vi "Offset Structure.vi"(10 "Structure Type":T1, 11 "MasterRect in":T2) -> (3 "MasterRect out":T2)   [LabVIEW 2020, in "Enclose in Structure.lvlib"]
uses:
  Enclose in Structure.lvlib
  <vilib>/Utility/miscctls.llb/LVRectTypeDef.ctl
  Structure Type.ctl
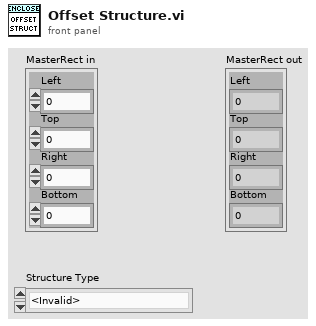
[diagram p1: front panel]
types:
  T1 = typedef "Enclose in Structure.lvlib/Structure Type.ctl" = enum16{"<Invalid>", "For Loop", "While Loop", "Timed Loop", "Timed Sequence", "Case Structure", "Event Structure", "In Place Element Structure", "Flat Sequence", "Diagram Disable Structure", "Conditional Disable Structure", "Type Specialization Structure"}
  T2 = typedef "LVRectTypeDef.ctl" = cluster{"Left":i16, "Top":i16, "Right":i16, "Bottom":i16}
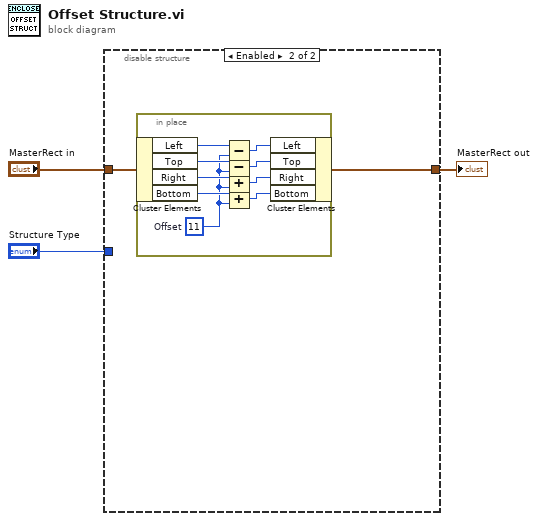
[diagram p0: block diagram]
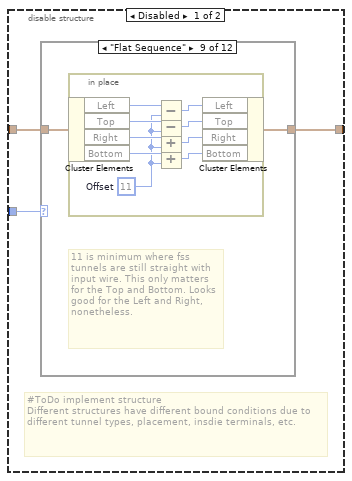
[diagram p2: hidden frame]
diagram:
  n1 = disable-structure shown="Enabled" {
    disable-tunnel: "MasterRect in" -> [w6 w30]
    disable-tunnel: [w5 w29] -> w2
    disable-tunnel: "Structure Type" -> [w4 _]
    frame Disabled {
      # "#ToDo implement structure\nDifferent structures have different bound conditions due to different tunnel types, placement, insdie terminals, etc."
      n2 = case shown="\"Flat Sequence\"" w4 {
        tunnel: w6 -> [w7 w8 w9 w10 w11 w12 w13 w14 w16 w26 w27 w28]
        tunnel: [w7 w8 w9 w10 w11 w12 w13 w14 w15 w26 w27 w28] -> w5
        frame "<Invalid>", Default {
          # "#davnat No-Op"
        }
        frame "For Loop" {
        }
        frame "While Loop" {
        }
        frame "Timed Loop" {
        }
        frame "Timed Sequence" {
        }
        frame "Case Structure" {
        }
        frame "Event Structure" {
        }
        frame "In Place Element Structure" {
        }
        frame "Flat Sequence" {
          # "11 is minimum where fss tunnels are still straight with input wire. This only matters for the Top and Bottom. Looks good for the Left and Right, nonetheless."
          n3 = in-place {
            w17 = i16 11  # Offset
            n4 = in-place-cluster #1(w16) -> ("Left"=w25:i16, "Top"=w24:i16, "Right"=w23:i16, "Bottom"=w22:i16)
            n5 = Subtract(x=w25, y=w17) -> (x-y=w21:i16)
            n6 = Subtract(x=w24, y=w17) -> (x-y=w20:i16)
            n7 = Add(x=w23, y=w17) -> (x+y=w19:i16)
            n8 = Add(x=w22, y=w17) -> (x+y=w18:i16)
            n9 = in-place-cluster #1("Left"=w21, "Top"=w20, "Right"=w19, "Bottom"=w18) -> (w15:T2)
          }
        }
        frame "Diagram Disable Structure" {
        }
        frame "Conditional Disable Structure" {
        }
        frame "Type Specialization Structure" {
        }
      }
    }
    frame Enabled {
      n10 = in-place {
        w31 = i16 11  # Offset
        n11 = in-place-cluster #2(w30) -> ("Left"=w39:i16, "Top"=w38:i16, "Right"=w37:i16, "Bottom"=w36:i16)
        n12 = Subtract(x=w39, y=w31) -> (x-y=w35:i16)
        n13 = Subtract(x=w38, y=w31) -> (x-y=w34:i16)
        n14 = Add(x=w37, y=w31) -> (x+y=w33:i16)
        n15 = Add(x=w36, y=w31) -> (x+y=w32:i16)
        n16 = in-place-cluster #2("Left"=w35, "Top"=w34, "Right"=w33, "Bottom"=w32) -> (w29:T2)
      }
    }
  }
  "MasterRect out" <- w2
